vi "test4_xcooruniform.vi"() -> ()   [LabVIEW 2018]
uses:
  <vilib>/imath/engines/lvmath2/RunTimeEngine/BuiltInFunctions/randnormal/NIMS_randnormal(1,I32).vi
  <vilib>/imath/engines/lvmath2/RunTimeEngine/ErrorHandling/NIMS_Error From Error Code.vi
  <vilib>/imath/engines/lvmath2/RunTimeEngine/BuiltInFunctions/crosscorr/NIMS_crosscorr(GM,Str).vi
  <instcachedir>/0/NIMS_crosscorr(GM,Str)_B40E69E1A515490ABE9B33FB59F56A52.lvgen/NIMS_crosscorr(GM,Str)_B40E69E1A515490ABE9B33FB59F56A52_001.vi
  <vilib>/imath/engines/lvmath2/RunTimeEngine/BuiltInFunctions/crosscorr/NIMS_crosscorr(GV,GV,Str).vi
  <instcachedir>/0/NIMS_crosscorr(GV,GV,Str)_A4EB815E9E924C97804DA22507CDE303.lvgen/NIMS_crosscorr(GV,GV,Str)_A4EB815E9E924C97804DA22507CDE303_000.vi
  <vilib>/imath/engines/lvmath2/RunTimeEngine/IndexRead/NIMS M(S,$).vi
  <instcachedir>/0/NIMS M(S,$)_F24F360562DE41D8BE234322A2E15C65.lvgen/NIMS M(S,$)_F24F360562DE41D8BE234322A2E15C65_001.vi
  <vilib>/imathl/engines/lvmath/Functions/Error Handling/Create Error.vi
  <vilib>/imath/engines/lvmath2/RunTimeEngine/NodeEndStatement/NIMS_NodeEndStatement_Output.vi
  <instcachedir>/0/NIMS_NodeEndStatement_Output_53EC0D466D134D7ABD903AC30B43404B.lvgen/NIMS_NodeEndStatement_Output_53EC0D466D134D7ABD903AC30B43404B_000.vi
  <instcachedir>/0/NIMS_NodeEndStatement_Output_53EC0D466D134D7ABD903AC30B43404B.lvgen/NIMS_NodeEndStatement_Output_53EC0D466D134D7ABD903AC30B43404B_005.vi
  <vilib>/imath/engines/lvmath2/RunTimeEngine/ErrorHandling/NIMS_Finalize Error.vi
panel:
  out "相关函数":cluster{"t":dbl[], "y":dbl[]}[](graph)
  in  "num":dbl=10000.0
  in  "a2":dbl=4.0
  in  "mn2":dbl=3.0
  in  "a1":dbl=2.0
  in  "mn1":dbl=1.0
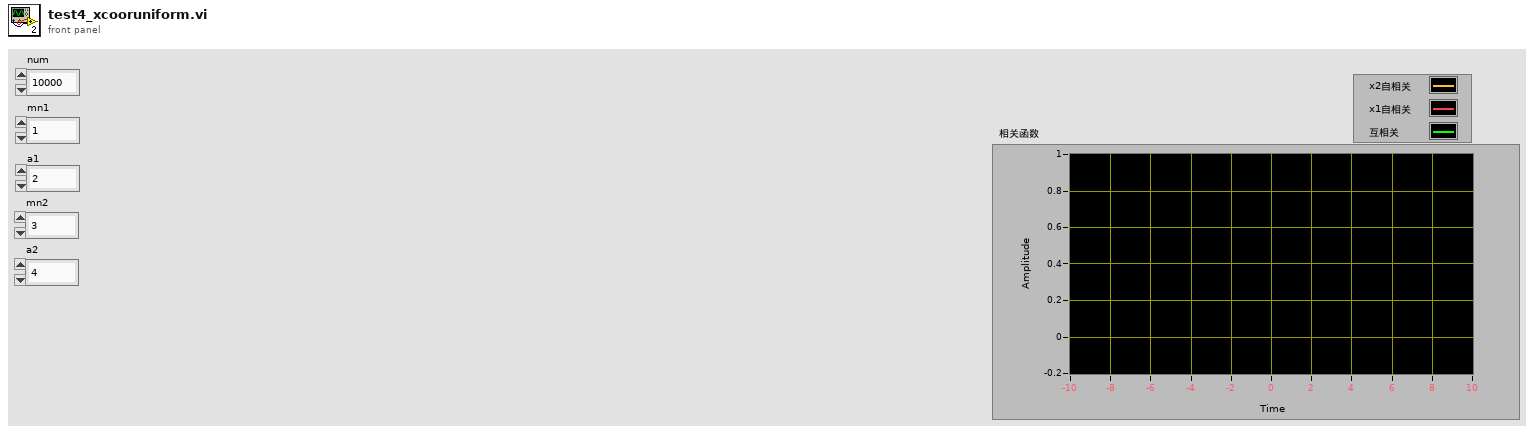
[diagram p1: front panel]
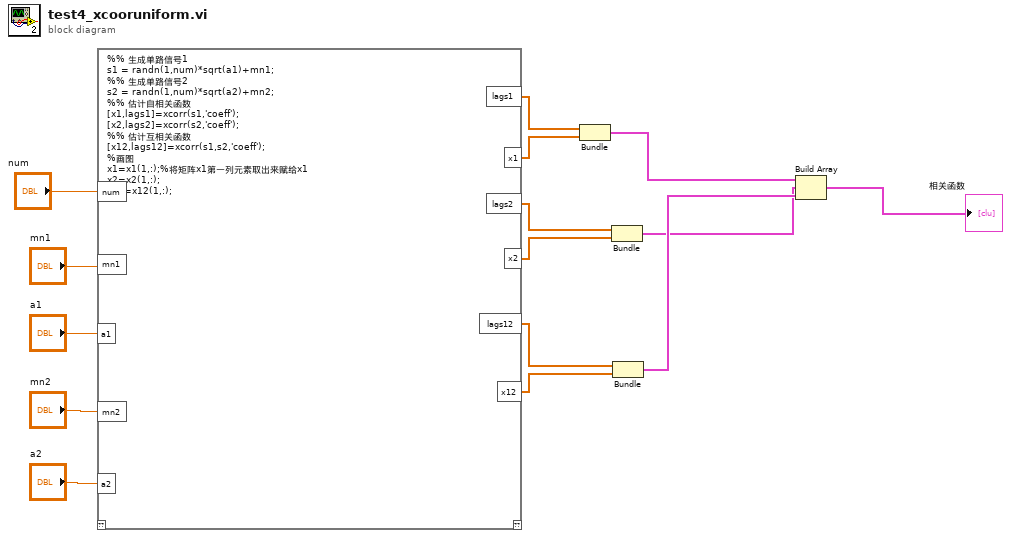
[diagram p0: block diagram]
diagram:
  n1 = mathscript code="%% 生成单路信号1\ns1 = randn(1,num)*sqrt(a1)+mn1;\n%% 生成单路信号2\ns2 = randn(1,num)*sqrt(a2)+mn2;\n%% 估计自相关函数\n[x1,lags1]=xcorr(s1,'coeff');\n[x2,lags2]=xcorr(s2,'coeff');\n%% 估计互相关函数\n[x12,lags12]=xcorr(s1,s2,'coeff');\n%画图\nx1=x1(1,:);%将矩阵x1第一列元素取出来赋给x1\nx2=x2(1,:);\nx12=x12(1,:);"("num"="num", "mn1"="mn1", "a1"="a1", "mn2"="mn2", "a2"="a2") -> ("lags1"=w11:dbl[], "x1"=w10:cdb[], "lags2"=w9:dbl[], "x2"=w8:cdb[], "lags12"=w7:dbl[], "x12"=w6:cdb[])  [unwired: 1 in, 1 out]
  n2 = Bundle("lags1"=w11, "x1"=w10) -> (w2:cluster{"lags1":dbl[], "x1":cdb[]})  [unwired: 1 in]
  n3 = Bundle("lags2"=w9, "x2"=w8) -> (w1:cluster{"lags2":dbl[], "x2":cdb[]})  [unwired: 1 in]
  n4 = Bundle("lags12"=w7, "x12"=w6) -> (w3:cluster{"lags12":dbl[], "x12":cdb[]})  [unwired: 1 in]
  n5 = Build Array(w2, w1, w3) -> (→"相关函数":cluster{"lags12":dbl[], "x12":cdb[]}[])
